vi "Data stream writer.vi"() -> ()   [LabVIEW 2015]
panel:
  out "Data stream writer":refnum<k21>
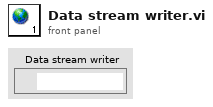
[diagram p1: front panel]
diagram:
